vi "Adjust for ROI.vi"(6 "wavelengths":dbl[](array[numeric]), 9 "X Length":i32, 10 "X Start":i32, 11 "X Binning":i32) -> (1 "subarray":dbl[](array[numeric]), 2 "Wavelengths":dbl[](array[numeric]), 3 "Ramp Pattern":dbl[](array[numeric]))   [LabVIEW 2019, in "Spectrometer Calibration.lvlib"]
uses:
  Spectrometer Calibration.lvlib
  <vilib>/Analysis/1siggen.llb/Ramp Pattern by Samples.vi
  <vilib>/Analysis/NI_AALBase.lvlib
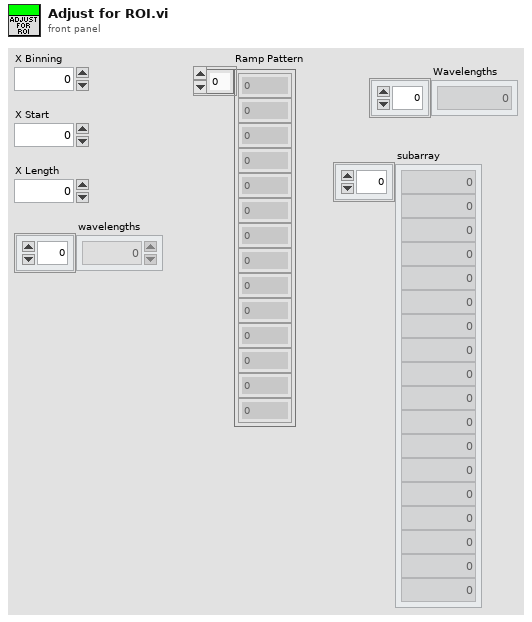
[diagram p1: front panel]
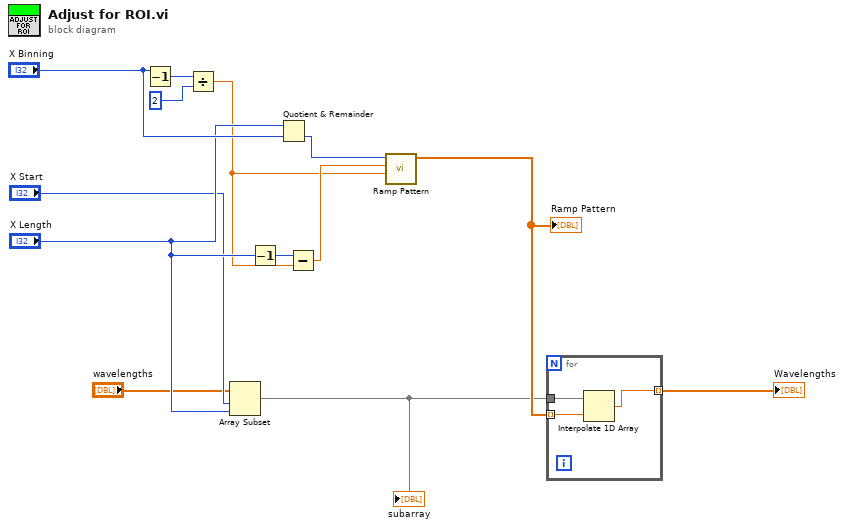
[diagram p0: block diagram]
diagram:
  n1 = Decrement(x="X Binning") -> (x-1=w3:i32)
  n2 = Divide(x=w3, y=2) -> (x/y=w5:dbl)
  n3 = Array Subset(array="wavelengths", index="X Start", length="X Length") -> (w7:dbl[])
  "subarray" <- w7
  n4 = Decrement(x="X Length") -> (x-1=w13:i32)
  n5 = Quotient & Remainder(x="X Length", y="X Binning") -> (floor(x/y)=w12:i32)  [unwired: 1 out]
  n6 = Subtract(x=w13, y=w5) -> (x-y=w6:dbl)
  n7 = call-poly <vilib>:"Ramp Pattern.vi"("start"=w5, "end"=w6, "samples"=w12) -> ("Ramp Pattern"=w8:dbl[])  [unwired: 7 in, 1 out]
  "Ramp Pattern" <- w8
  n8 = for {
    tunnel: w7 -> [w16]
    tunnel: w8 -> [w15] mode=indexing
    tunnel: [w14] -> w9 mode=indexing
    n9 = Interpolate 1D Array(1:w15, 2:w16) -> (0:w14:dbl)
  }
  "Wavelengths" <- w9
